vi "Finish.vi"   [LabVIEW 2011]
doc: "This VI is called just before exiting. It is expected to close I/O refnum, save collected data, etc."
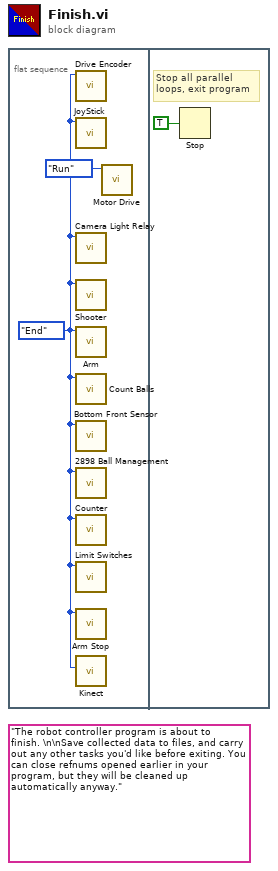
[diagram p0: block diagram]
diagram:
  (unwired) "The robot controller program is about to finish. \n\nSave collected data to files, and carry out any other tasks you'd like before exiting. You can close refnums opened earlier in your program, but they will be cleaned up automatically anyway."
  n1 = flat-sequence {
    frame #0 {
      w2 = enum16{"Init", "Run", "End"}."End" ("Enum")
      n2 = call "Drive Encoder.vi"("Enum"=w2) -> ()  [unwired: 10 in, 1 out]
      n3 = call "JoyStick.vi"("Enum"=w2) -> ()  [unwired: 7 in, 4 out]
      n4 = call "Camera Light Relay.vi"("Enum"=w2) -> ()  [unwired: 11 in]
      n5 = call "Shooter.vi"("Enum"=w2) -> ()  [unwired: 10 in]
      n6 = call "Arm.vi"("Enum"=w2) -> ()  [unwired: 11 in]
      n7 = call "Count Balls.vi"("Mode"=w2) -> ()  [unwired: 8 in, 3 out]
      n8 = call "Bottom Front Sensor.vi"("Enum"=w2) -> ()  [unwired: 10 in, 1 out]
      n9 = call "2898 Ball Management.vi"("Enum"=w2) -> ()  [unwired: 11 in]
      n10 = call "Counter.vi"("Enum"=w2) -> ()  [unwired: 10 in, 1 out]
      n11 = call "Limit Switches.vi"("Enum"=w2) -> ()  [unwired: 9 in, 2 out]
      n12 = call "Arm Stop.vi"("Enum"=w2) -> ()  [unwired: 10 in]
      n13 = call "Kinect.vi"("Mode"=w2) -> ()  [unwired: 10 in, 1 out]
      n14 = call "Motor Drive.vi"("Enum"=enum16{"Init", "Run", "SetBrakeCoast", "End"}."Run") -> ()  [unwired: 11 in]
    }
    frame #1 {
      # "Stop all parallel\nloops, exit program"
      n15 = Stop(stop? (T)=TRUE ("Quit")) -> ()
    }
  }
